vi "testETPA&TPA.vi"() -> ()   [LabVIEW 2023]
panel:
  in  "number of measurements":i32
  out "number of measurements":i32
  in  "speed of taking measurments 2":u32
  out "break time ms 2":u32=100
  out "Collection Time 2":u32=1000
  out "Function (1: AC Volts)\nFunction(0: DC Volts)":u16=1
  out "counter  2":tag="Dev1/ctr0"
  out "source  2":tag="/Dev1/PFI14"
  out "VISA resource name mulitmeter  2":refnum<visa-resource-name>="sarasMultimeter"
  in  "VISA resource name mulitmeter":refnum<visa-resource-name>
  in  "DEFAULT?":bool
  in  "Collection Time":u32
  in  "Label?":bool
  in  "Wavescan?":bool
  in  "file path (dialog if empty)":path
  in  "?":bool
  out "PRESENT - COUNTER":dbl(graph)
  out "PRESENT - Multimeter":dbl(graph)
  in  "Function (1: AC Volts)\nFunction(0: DC Volts)":u16
  in  "break time ms":u32
  in  "source":tag
  in  "counter":tag
  out "Current Trial -Multimeter":dbl(graph)
  out "Current Trial - Singles Photon Count Rate":dbl(graph)
  in  "speed of taking measurments":u32
  # "Default Settings"
  # "CTR0"
  # "USB0"
  # "PFI14"
  # "Not Default Settings"
  # "PLEASE PUT (\".csv\") at the end of your path"
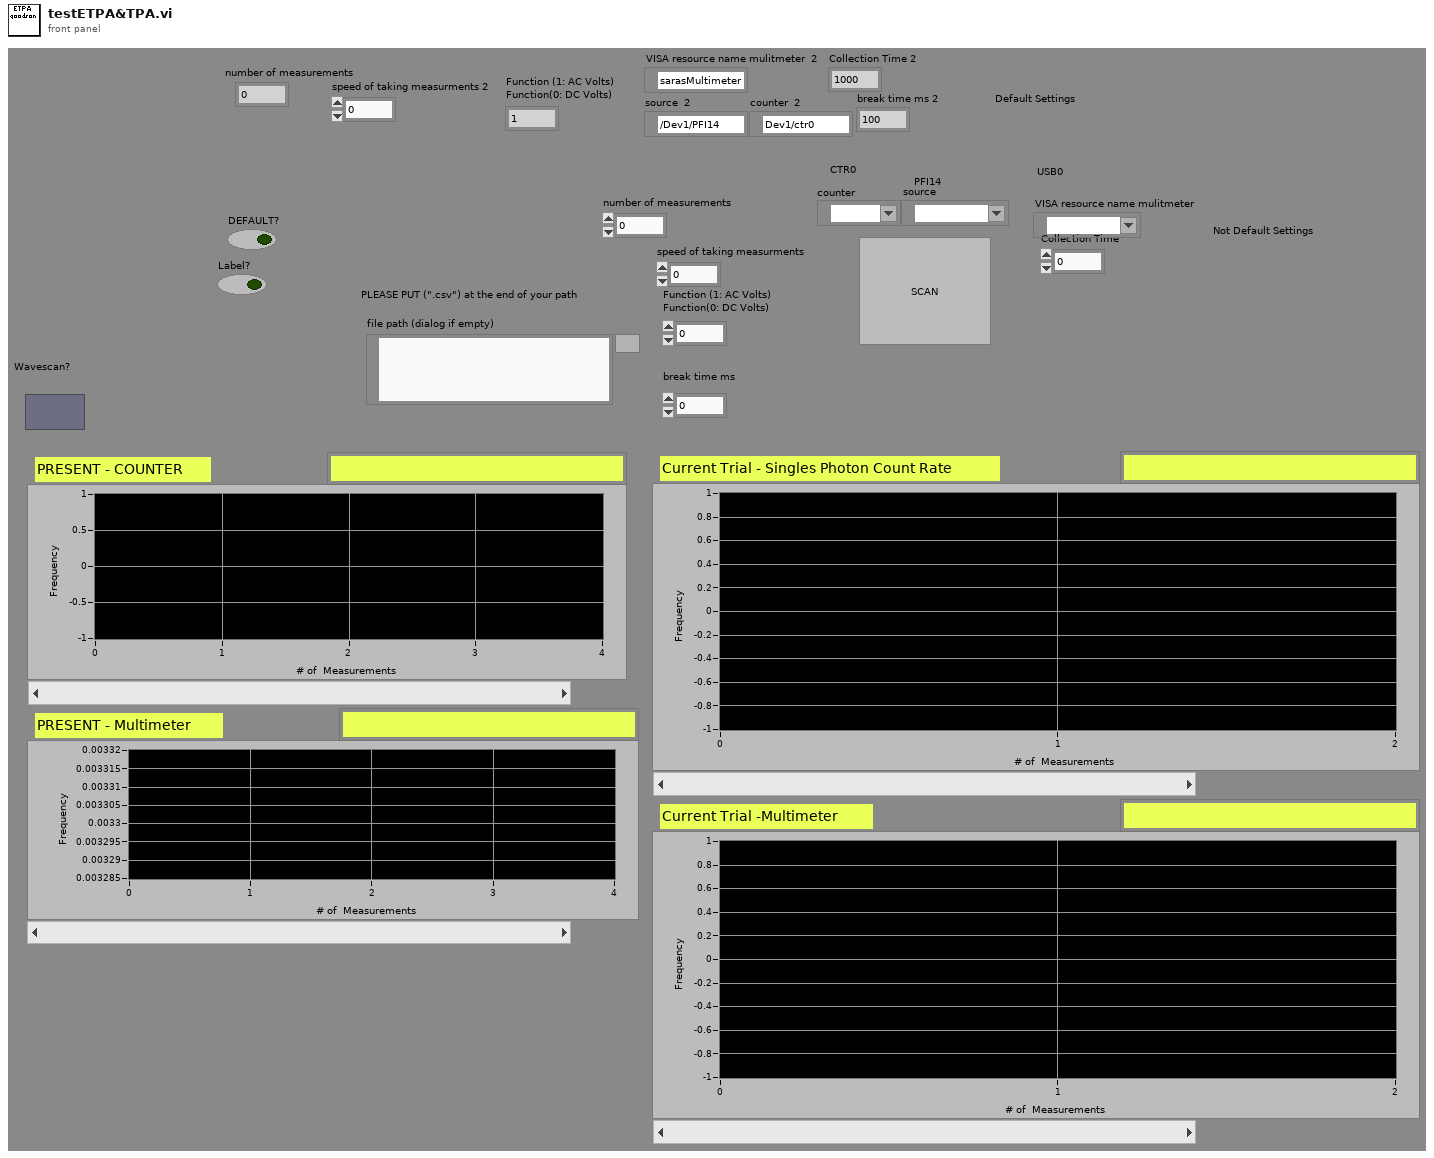
[diagram p1: front panel]
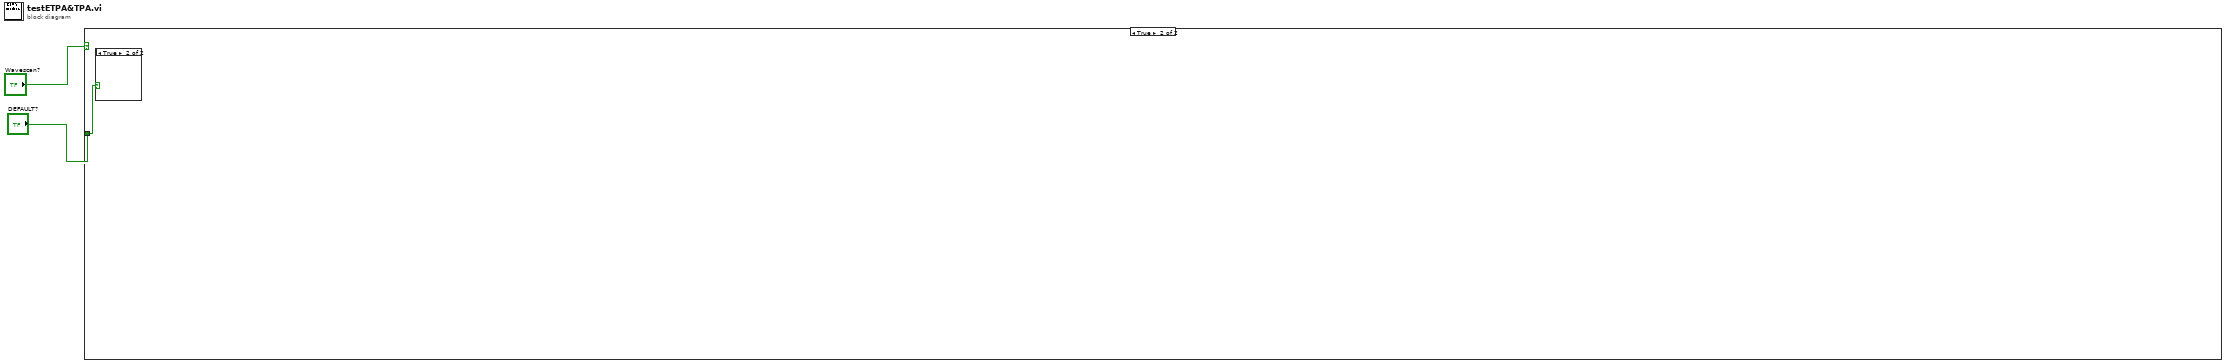
[diagram p0: block diagram]
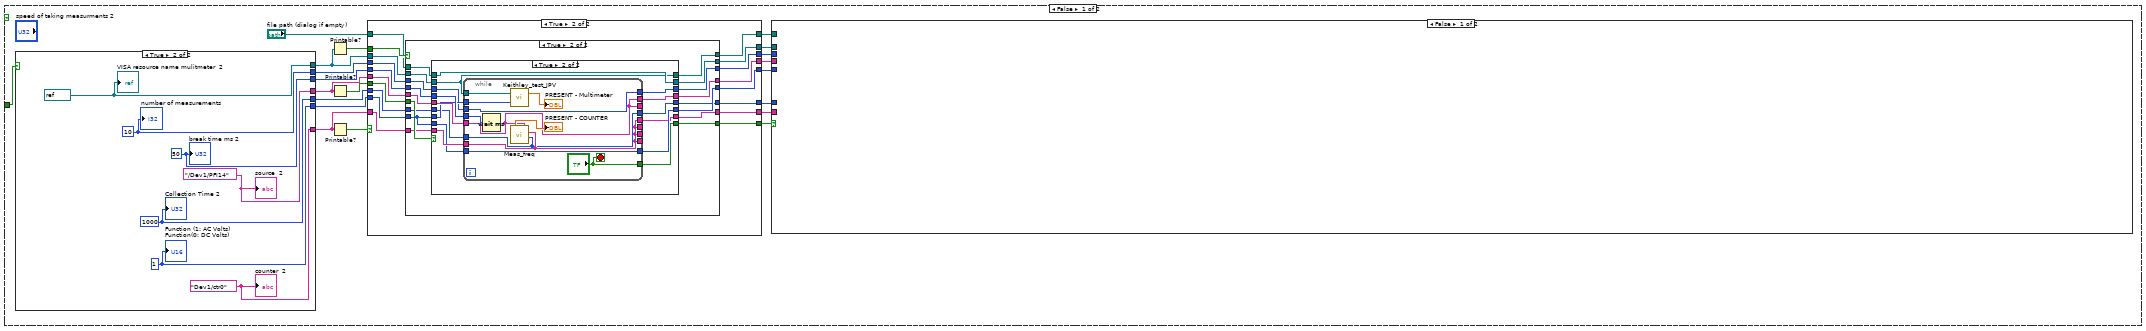
[diagram p2: hidden frame]
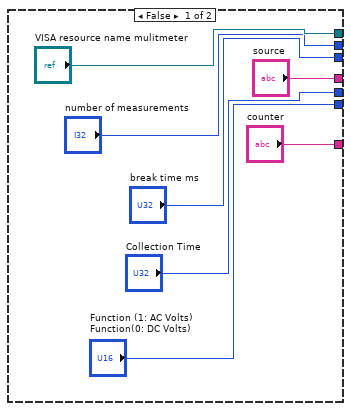
[diagram p3: hidden frame]
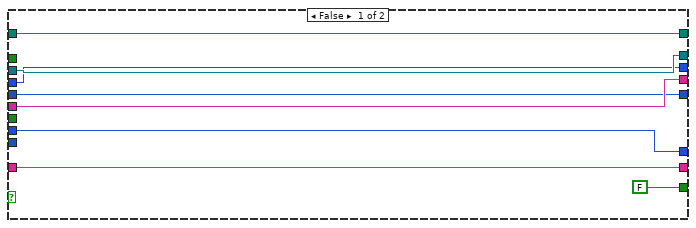
[diagram p4: hidden frame]
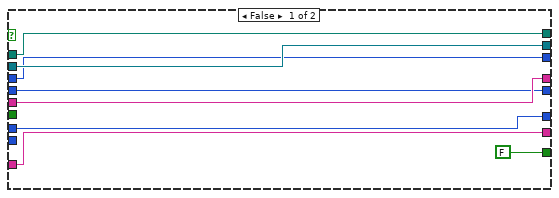
[diagram p5: hidden frame]
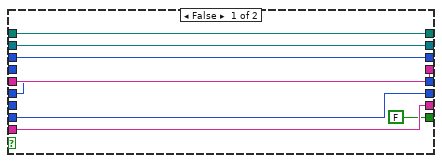
[diagram p6: hidden frame]
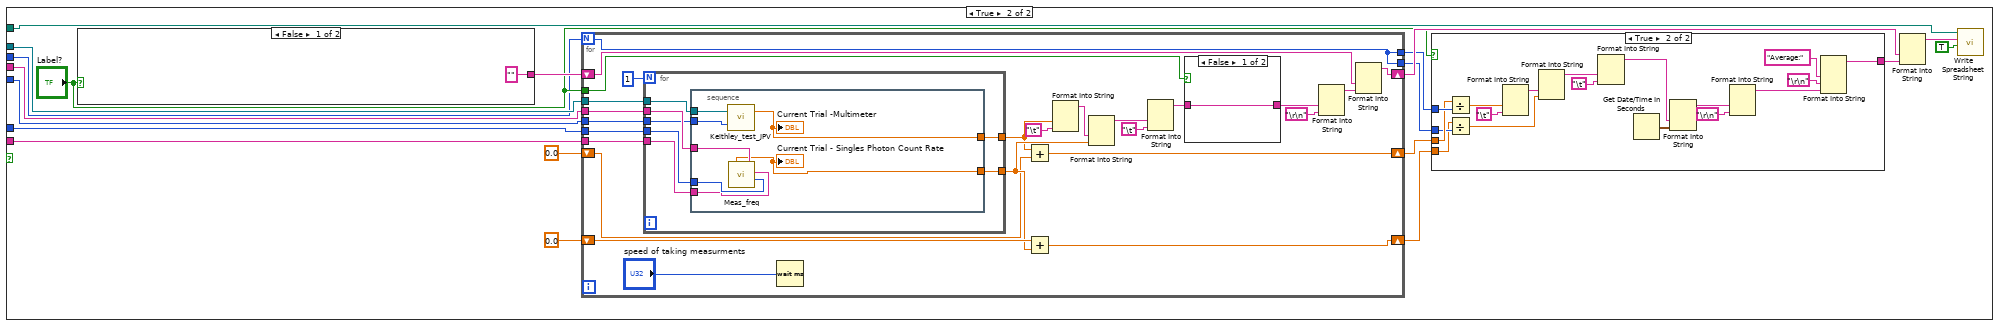
[diagram p7: hidden frame]
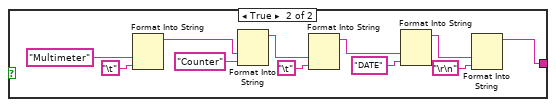
[diagram p8: hidden frame]
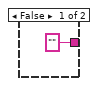
[diagram p9: hidden frame]
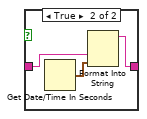
[diagram p10: hidden frame]
diagram:
  n1 = case shown="True" "Wavescan?" {
    tunnel: "DEFAULT?" -> [w5 w215]
    frame False {
      n2 = case shown="True" w5 {
        tunnel: ["VISA resource name mulitmeter" w36] -> w11
        tunnel: ["break time ms" w35] -> w10
        tunnel: ["Collection Time" w34] -> w9
        tunnel: ["Function (1: AC Volts)\nFunction(0: DC Volts)" w33] -> w8
        tunnel: ["source" w32] -> w7
        tunnel: ["counter" w31] -> w6
        tunnel: ["number of measurements" w30] -> w3
        frame False {
        }
        frame True {
          w30 = 10
          w31 = tag "Dev1/ctr0" ("counter")
          w32 = tag "/Dev1/PFI14" ("source")
          w33 = u16 1 ("Function (1: AC Volts)\nFunction(0: DC Volts)")
          w34 = u32 1000 ("Collection Time")
          w35 = u32 50 ("break time ms")
          w36 = refnum<visa-resource-name> "BO" ("VISA resource name mulitmeter")
          "VISA resource name mulitmeter  2" <- w36
          "source  2" <- w32
          "counter  2" <- w31
          "Function (1: AC Volts)\nFunction(0: DC Volts)" <- w33
          "Collection Time 2" <- w34
          "break time ms 2" <- w35
          "number of measurements" <- w30
        }
      }
      n3 = Printable?(1:w11) -> (0:w13:bool)
      n4 = Printable?(1:w7) -> (0:w12:bool)
      n5 = Printable?(1:w6) -> (0:w14:bool)
      n6 = case shown="True" w14 {
        tunnel: w13 -> [_ w62]
        tunnel: w12 -> [_ w61]
        tunnel: w6 -> [w41 w60]
        tunnel: w11 -> [w39 w59]
        tunnel: w7 -> [w42 w58]
        tunnel: w10 -> [w40 w57]
        tunnel: w8 -> [_ w56]
        tunnel: [w42 w55] -> w22
        tunnel: [w39 w54] -> w21
        tunnel: [w40 w53] -> w20
        tunnel: [w41 w52] -> w19
        tunnel: [FALSE w51] -> w18
        tunnel: [w44 w50] -> w17
        tunnel: [w38 w49] -> w16
        tunnel: "file path (dialog if empty)" -> [w44 w48]
        tunnel: w9 -> [w38 w47]
        tunnel: w3 -> [w37 w46]
        tunnel: [w37 w45] -> w4
        frame False {
        }
        frame True {
          n7 = case shown="True" w62 {
            tunnel: w61 -> [_ w87]
            tunnel: w60 -> [w68 w86]
            tunnel: w59 -> [w67 w85]
            tunnel: w58 -> [w70 w84]
            tunnel: w57 -> [w69 w83]
            tunnel: w56 -> [_ w82]
            tunnel: [w70 w81] -> w55
            tunnel: [w67 w80] -> w54
            tunnel: [w69 w79] -> w53
            tunnel: [w68 w78] -> w52
            tunnel: [FALSE w77] -> w51
            tunnel: [w65 w76] -> w50
            tunnel: [w64 w75] -> w49
            tunnel: w48 -> [w65 w74]
            tunnel: w47 -> [w64 w73]
            tunnel: w46 -> [w63 w72]
            tunnel: [w63 w71] -> w45
            frame False {
            }
            frame True {
              n8 = case shown="True" w87 {
                tunnel: [w94 w105] -> w81
                tunnel: [w95 w104] -> w80
                tunnel: [w92 w108] -> w79
                tunnel: [w93 w106] -> w78
                tunnel: [FALSE w103] -> w77
                tunnel: [w90 w99] -> w76
                tunnel: [w89 w107] -> w75
                tunnel: w86 -> [w93 w109]
                tunnel: w85 -> [w95 w104]
                tunnel: w84 -> [w94 w110]
                tunnel: w83 -> [_ w102]
                tunnel: w82 -> [w92 w101]
                tunnel: w82 -> [_ w100]
                tunnel: w74 -> [w90 w99]
                tunnel: w73 -> [w89 w98]
                tunnel: w72 -> [w88 w97]
                tunnel: [w88 w96] -> w71
                frame False {
                }
                frame True {
                  n9 = while {
                    tunnel: [w116] -> w108
                    tunnel: [w114] -> _
                    tunnel: [w113] -> w107
                    tunnel: [w114] -> _
                    tunnel: [w114] -> _
                    tunnel: [w112] -> _
                    tunnel: w104 -> [w119]
                    tunnel: w110 -> [w112]
                    tunnel: w109 -> [w114]
                    tunnel: [w114] -> w106
                    tunnel: [w112] -> w105
                    tunnel: ["?"] -> w103
                    tunnel: w102 -> [w117]
                    tunnel: w101 -> [w116]
                    tunnel: w100 -> [w115]
                    tunnel: w98 -> [w113]
                    tunnel: w97 -> [w111]
                    tunnel: [w111] -> w96
                    stop <- "?" stop-if-true
                    n10 = Wait (ms)(milliseconds to wait=w117) -> ()  [unwired: 1 out]
                    n11 = call "Keithley_test_JPV.vi"("Function (0: DC Volts)"=w115, "VISA resource name"=w119) -> ("Measurement"=→"PRESENT - Multimeter":dbl)  [unwired: 1 out]
                    n12 = call "Meas_freq.vi"("source"=w112, "counter"=w114, "Time miliseconds"=w113) -> (0:→"PRESENT - COUNTER":dbl)  [unwired: 1 in]
                  }
                }
              }
            }
          }
        }
      }
      n13 = case shown="False" w18 {
        tunnel: w16 -> [_ w140]
        tunnel: w22 -> [_ w139]
        tunnel: w21 -> [_ w138]
        tunnel: w20 -> [_ w137]
        tunnel: w19 -> [_ w136]
        tunnel: w17 -> [_ w135]
        tunnel: w4 -> [_ w122]
        frame False {
        }
        frame True {
          n14 = case shown="False" "Label?" {
            tunnel: ["" w147] -> w134
            frame False {
            }
            frame True {
              n15 = Format Into String("Multimeter" ("input 2"), "\t") -> (resulting string=w151:string)  [unwired: 3 in, 1 out]
              n16 = Format Into String(w151, "Counter" ("input 2")) -> (resulting string=w146:string)  [unwired: 3 in, 1 out]
              n17 = Format Into String(w146, "\t") -> (resulting string=w144:string)  [unwired: 3 in, 1 out]
              n18 = Format Into String(w144, "DATE" ("input 2")) -> (resulting string=w143:string)  [unwired: 3 in, 1 out]
              n19 = Format Into String(w143, "\r\n") -> (resulting string=w147:string)  [unwired: 3 in, 1 out]
            }
          }
          n20 = for {
            N: w122 -> [w189]
            tunnel: w140 -> [w196]
            tunnel: w139 -> [w195]
            tunnel: w138 -> [w194]
            tunnel: w137 -> [w193]
            tunnel: w136 -> [w192]
            shift-right: [w190] -> w133
            shift-left: w134 -> [w191]
            shift-right: [w174] -> w124
            shift-left: 0.0 -> [w179]
            shift-right: [w175] -> w126
            shift-left: 0.0 -> [w176]
            tunnel: [w189] -> w125
            tunnel: [w189] -> w127
            tunnel: "Label?" -> [w173]
            n21 = for {
              N: 1 -> [_]
              tunnel: w196 -> [w207]
              tunnel: w195 -> [w206]
              tunnel: w194 -> [w205]
              tunnel: w193 -> [w204]
              tunnel: w192 -> [w203]
              tunnel: [w202] -> w177
              tunnel: [w201] -> w178
              n22 = stacked-sequence {
                tunnel: w207 -> [w214]
                tunnel: w206 -> [w213]
                tunnel: w205 -> [w212]
                tunnel: w204 -> [w211]
                tunnel: w203 -> [w208]
                tunnel: [w210] -> w202
                tunnel: [w209] -> w201
                frame #0 {
                  n23 = call "Keithley_test_JPV.vi"("Function (0: DC Volts)"=w211, "VISA resource name"=w212) -> ("Measurement"=w210:dbl)  [unwired: 1 out]
                  "Current Trial -Multimeter" <- w210
                  n24 = call "Meas_freq.vi"("source"=w213, "counter"=w208, "Time miliseconds"=w214) -> (0:w209:dbl)  [unwired: 1 in]
                  "Current Trial - Singles Photon Count Rate" <- w209
                }
              }
            }
            n25 = Wait (ms)(milliseconds to wait="speed of taking measurments") -> ()  [unwired: 1 out]
            n26 = Add(x=w177, y=w176) -> (x+y=w175:dbl)
            n27 = Add(x=w179, y=w178) -> (x+y=w174:dbl)
            n28 = Format Into String(w177, "\t") -> (resulting string=w183:string)  [unwired: 3 in, 1 out]
            n29 = Format Into String(w183, w178) -> (resulting string=w185:string)  [unwired: 3 in, 1 out]
            n30 = Format Into String(w185, "\t") -> (resulting string=w186:string)  [unwired: 3 in, 1 out]
            n31 = case shown="False" w173 {
              tunnel: [w197 w200] -> w187
              tunnel: w186 -> [w197 w199]
              frame False {
              }
              frame True {
                n32 = Get Date/Time In Seconds() -> (seconds since 1Jan1904=w198:timestamp)
                n33 = Format Into String(w199, w198) -> (resulting string=w200:string)  [unwired: 3 in, 1 out]
              }
            }
            n34 = Format Into String(w187, "\r\n") -> (resulting string=w184:string)  [unwired: 3 in, 1 out]
            n35 = Format Into String(w191, w184) -> (resulting string=w190:string)  [unwired: 3 in, 1 out]
          }
          n36 = case shown="True" "Label?" {
            tunnel: ["" w165] -> w128
            tunnel: w127 -> [_ w159]
            tunnel: w126 -> [_ w158]
            tunnel: w125 -> [_ w156]
            tunnel: w124 -> [_ w155]
            frame False {
            }
            frame True {
              n37 = Divide(x=w158, y=w159) -> (x/y=w157:dbl)
              n38 = Divide(x=w155, y=w156) -> (x/y=w154:dbl)
              n39 = Format Into String(w157, "\t") -> (resulting string=w164:string)  [unwired: 3 in, 1 out]
              n40 = Format Into String(w164, w154) -> (resulting string=w163:string)  [unwired: 3 in, 1 out]
              n41 = Format Into String(w163, "\t") -> (resulting string=w160:string)  [unwired: 3 in, 1 out]
              n42 = Get Date/Time In Seconds() -> (seconds since 1Jan1904=w169:timestamp)
              n43 = Format Into String(w160, w169) -> (resulting string=w171:string)  [unwired: 3 in, 1 out]
              n44 = Format Into String(w171, "\r\n") -> (resulting string=w166:string)  [unwired: 3 in, 1 out]
              n45 = Format Into String("Average:" ("input 4"), "\r\n", w166) -> (resulting string=w165:string)  [unwired: 3 in, 1 out]
            }
          }
          n46 = Format Into String(w133, w128) -> (resulting string=w129:string)  [unwired: 3 in, 1 out]
          n47 = call <vilib>:"Write Spreadsheet String.vi"("append to file? (new file:F)"=TRUE, "spreadsheet string"=w129, "file path (dialog if empty)"=w135) -> ()  [unwired: 7 in, 2 out]
        }
      }
    }
    frame True {
      n48 = case shown="True" w215 {
        frame False {
        }
        frame True {
        }
      }
    }
  }
